vi "New Query Template.vi"   [LabVIEW 2020, in "Application.lvlib"]
uses:
  Application.lvlib
  Globals.vi
  Data Manager/Data Manager.lvclass
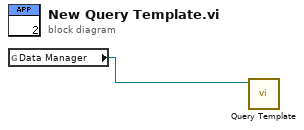
[diagram p0: block diagram]
diagram:
  n1 = global read "Globals.vi" "Data Manager"() -> (w1:refnum<class "Data Manager.lvclass">)
  n2 = call-dynamic "Query Template.vi"("Data Manager in"=w1) -> ()  [unwired: 9 in, 2 out]
